vi "poly VI B.vi"() -> ()   [LabVIEW 2009]
panel:
  in  "Cluster":cluster{"String":string, "Numeric":dbl}
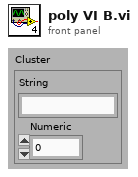
[diagram p1: front panel]
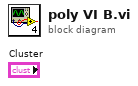
[diagram p0: block diagram]
diagram:
